vi "LU20_T_Control.vi"() -> ()   [LabVIEW 2013]
uses:
  Termo/1.5_16_ch_tango/tango_vi.llb/avToDoubleScalar.vi
  Termo/1.5_16_ch_tango/tango_vi.llb/tango.lvlib
panel:
  out "attribute names":string[](array[string])=["T1", "T2", "T3", "T4", "T5"]
  in  "stop":bool
  out "Напор \nобщий":dbl
  out "Cлив \nобщий":dbl
  out "K3":dbl
  out "К2":dbl
  out "К1":dbl
  out "Последнее обновление :":string
  out "Статус прибора":u32(colorbox) caption="ON"
  out "Tango device name":string="lu20/oil_termo/oil"
  # "Система охлаждения квадрупольных линз"
  # "ЛУ-20"
  # "°С"
  # "°С"
  # "°С"
  # "°С"
  # "°С"
  # "Бак \nтеплообменника"
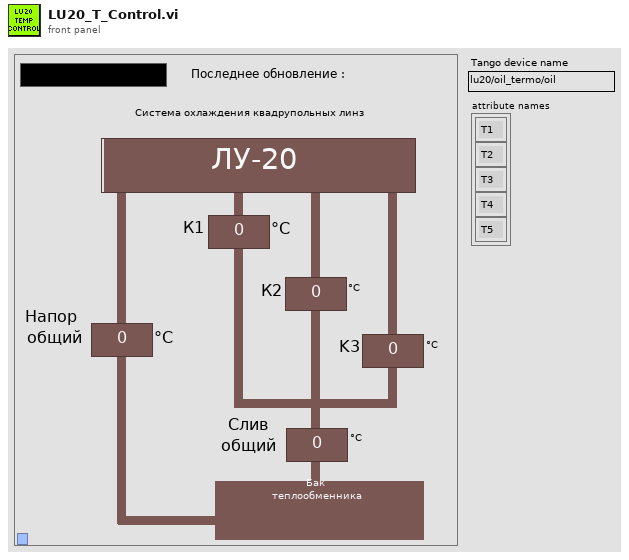
[diagram p1: front panel]
types:
  T1 = cluster{"device name":string, "attribute name":string, "quality value":i16, "quality string":string, "timestamp":dbl, "dim. x":i32, "dim. y":i32, "value":u8[], "error code":i32, "error stack":string[], "data type":u16}[]
  T2 = cluster{"device name":string, "attribute name":string, "quality value":i16, "quality string":string, "timestamp":dbl, "dim. x":i32, "dim. y":i32, "value":u8[], "error code":i32, "error stack":string[], "data type":u16}
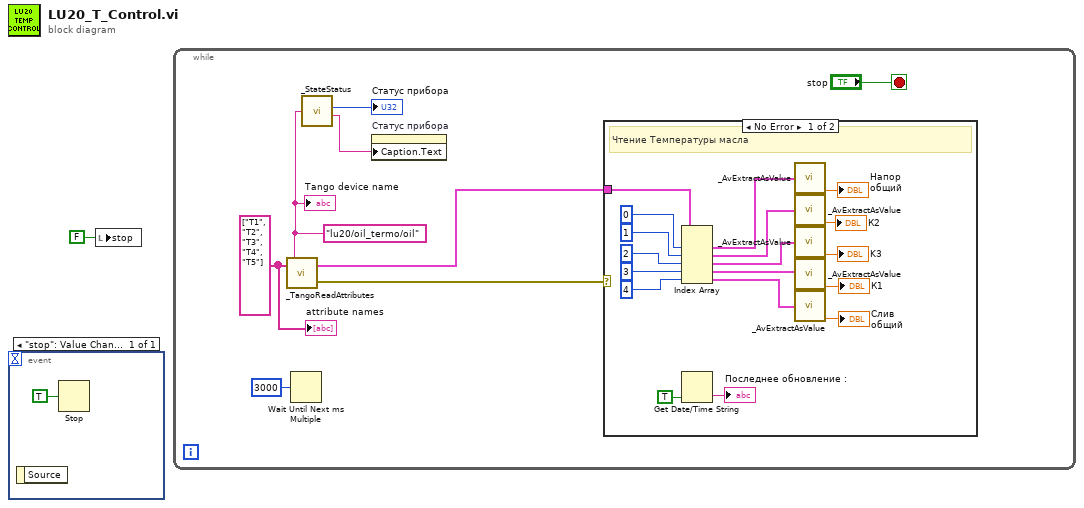
[diagram p0: block diagram]
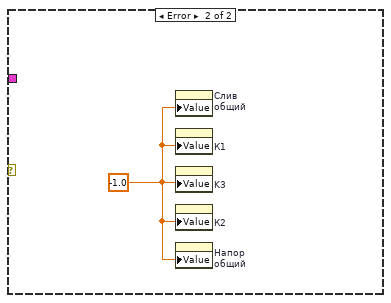
[diagram p2: hidden frame]
diagram:
  n1 = event shown="[0] \"stop\": Value Change" {
    selector: _ -> [_]
    dyn-events: _ -> [_]
    timeout: _ -> [_]
    event "stop": Value Change {
      n2 = event-data() -> ()  [unwired: 1 in, 1 out]
      n3 = Stop(stop? (T)=TRUE) -> ()
    }
  }
  n4 = local write "stop"(FALSE ("Boolean")) -> ()
  n5 = while {
    stop <- "stop" stop-if-true
    w5 = "lu20/oil_termo/oil" ("device name")
    w3 = string[] ["T1", "T2", "T3", "T4", "T5"] ("attribute names")
    n6 = call "_TangoReadAttributes.vi"("attribute names"=w3, "device name"=w5) -> ("error out"=w7:errorcluster, "attribute values"=w6:T1)  [unwired: 1 in]
    n7 = Wait Until Next ms Multiple(millisecond multiple=u32 3000) -> ()  [unwired: 1 out]
    n8 = call "_StateStatus.vi"("Device Name"=w5) -> ("State Color"=→"Статус прибора":u32, "State String"=w8:string)  [unwired: 4 out]
    n9 = property on="Статус прибора" class="ColBox"("Caption.Text"=w8) -> ()  [unwired: 2 in, 2 out]
    n10 = case shown="No Error" w7 {
      tunnel: w6 -> [w27 _]
      frame No Error {
        # "Чтение Температуры масла"
        n11 = Index Array(array=w27, index #1=0 ("indice"), index #2=1 ("index"), index #3=2 ("indice"), index #4=3 ("index"), index #5=4 ("index")) -> (element #1=w26:T2, element #2=w21:T2, element #3=w20:T2, element #4=w19:T2, element #5=w18:T2)
        n12 = Get Date/Time String(want seconds? (F)=TRUE) -> (time string=→"Последнее обновление :":string)  [unwired: 2 in, 1 out]
        n13 = call-poly "_AvExtractAsValue.vi"("attribute value"=w26) -> ("value"=→"Напор \nобщий":dbl)  [unwired: 4 out]
        n14 = call-poly "_AvExtractAsValue.vi"("attribute value"=w21) -> ("value"=→"К2":dbl)  [unwired: 4 out]
        n15 = call-poly "_AvExtractAsValue.vi"("attribute value"=w20) -> ("value"=→"K3":dbl)  [unwired: 4 out]
        n16 = call-poly "_AvExtractAsValue.vi"("attribute value"=w19) -> ("value"=→"К1":dbl)  [unwired: 4 out]
        n17 = call-poly "_AvExtractAsValue.vi"("attribute value"=w18) -> ("value"=→"Cлив \nобщий":dbl)  [unwired: 4 out]
      }
      frame Error {
        w29 = -1.0 ("millisecond multiple")
        n18 = property on="Cлив \nобщий" class="DigNum (strict)"("Value"=w29) -> ()  [unwired: 2 in, 2 out]
        n19 = property on="К1" class="DigNum (strict)"("Value"=w29) -> ()  [unwired: 2 in, 2 out]
        n20 = property on="K3" class="DigNum (strict)"("Value"=w29) -> ()  [unwired: 2 in, 2 out]
        n21 = property on="К2" class="DigNum (strict)"("Value"=w29) -> ()  [unwired: 2 in, 2 out]
        n22 = property on="Напор \nобщий" class="DigNum (strict)"("Value"=w29) -> ()  [unwired: 2 in, 2 out]
      }
    }
    "Tango device name" <- w5
    "attribute names" <- w3
  }
